vi "move_forvard.vi"(1 "output cluster":T1) -> (0 "action":T2)   [LabVIEW 2015, in "PolyVIEW.lvclass"]
uses:
  PolyVIEW.lvclass
  ant_base/action_cluster.ctl
  ant_base/actionType_enum.ctl
  Memory.ctl
  ant_base/ant_base.lvclass
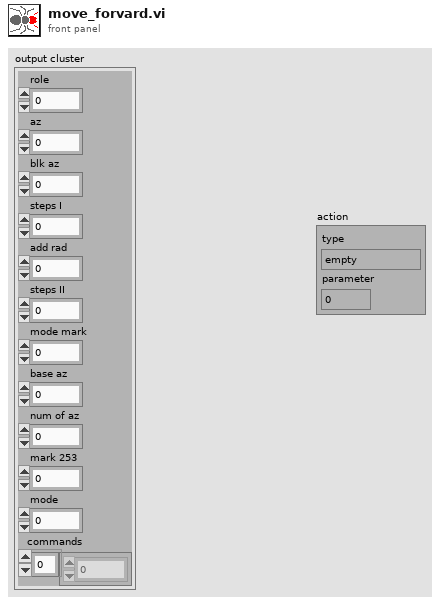
[diagram p1: front panel]
types:
  T1 = typedef "PolyVIEW.lvclass/Memory.ctl" = cluster{"role":i32, "az":i32, "blk az":i32, "steps I":u32, "add rad":i32, "steps II":u32, "mode mark":u32, "base az":u32, "num of az":u32, "mark 253":u32, "mode":u32, "commands":i32[]}
  T2 = typedef "ant_base.lvclass/action_cluster.ctl" = cluster{"type":T3, "parameter":dbl}
  T3 = typedef "ant_base.lvclass/actionType_enum.ctl" = enum8{"empty", "move", "take", "put", "mark"}
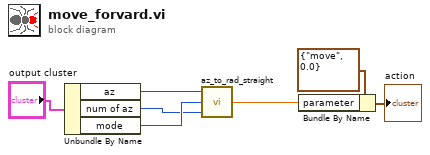
[diagram p0: block diagram]
diagram:
  n1 = Unbundle By Name("output cluster") -> ("az"=w3:i32, "num of az"=w2:u32, "mode"=w4:u32)
  n2 = call "az_to_rad_straight.vi"("az quantity"=w2, "mode"=w4, "az"=w3) -> ("rad"=w1:dbl)
  n3 = Bundle By Name(cluster=T2 {"type"=enum."move", "parameter"=0.0} ("action"), "parameter"=w1) -> (→"action":T2)
